vi "PicoScope2000ExampleBlockAdvancedTrigger.vi"() -> ()   [LabVIEW 2010]
uses:
  shared/PicoBuffers.ctl
  shared/Buffer and Transfer Settings.ctl
  shared/Acquisition Settings.ctl
  PicoScope2000Lib/PicoScope2000AnalogChannelSettings.ctl
panel:
  in  "Write to TDMS":bool
  in  "roundFaster":bool=TRUE
  in  "timeIntervalRequested":dbl min=0.0 format="%#6_6p"
  in  "Trigger Conditions":T1 {"PWQ" items=["Don't Care", "True", "False"]; "Ext" items=["Don't Care", "True", "False"]; "Channel D" items=["Don't Care", "True", "False"]; "Channel C" items=["Don't Care", "True", "False"]; "Channel B" items=["Don't Care", "True", "False"]; "Channel A" items=["Don't Care", "True", "False"]; "Condition Logic" items=["AND", "OR", "XOR"]}
  in  "Channel A Trigger Properties":T2={"thresholdUpper"=0, "thresholdHysteresis"=512, "thresholdLower"=0, "Threshold Mode"=0, "Direction"=2, "Available"=TRUE} {"Direction" items=["Above / Inside", "Below / Outside", "Rising / Enter", "Falling / Exit", "Rising or Falling / Enter or Exit", "Above Lower", "Below Lower", "Rising Lower", "Falling Lower", "Positive Runt", "Negative Runt"]; "Threshold Mode" items=["Level", "Window"]}
  in  "Pulse Width Qualifier Settings":T3={"Direction"=2, "Lower Limit"=0, "Upper Limit"=0, "Pulse Width Type"=0} {"Pulse Width Type" items=["None", "Less Than", "Greater Than", "In Range", "Out of Range"]; "Direction" items=["Rising"=2, "Falling"=3]}
  in  "Pulse Width Qualifier Conditions":T4 {"Condition Logic" items=["AND", "OR", "XOR"]}
  in  "Auto Trigger (ms)":i32=1000
  in  "Trigger Delay":u32
  in  "Channel B Settings":T5={"Enabled"=TRUE, "Coupling"=1, "Range"=6} {"Range" items=["20 mV"=1, "50 mV"=2, "100 mV"=3, "200 mV"=4, "500 mV"=5, "1 V"=6, "2 V"=7, "5 V"=8, "10 V"=9, "20 V"=10]; "Coupling" items=["AC", "DC"]}
  in  "Channel A Settings":T5={"Enabled"=TRUE, "Coupling"=1, "Range"=6} {"Range" items=["20 mV"=1, "50 mV"=2, "100 mV"=3, "200 mV"=4, "500 mV"=5, "1 V"=6, "2 V"=7, "5 V"=8, "10 V"=9, "20 V"=10]; "Coupling" items=["AC", "DC"]}
  out "Unit Info":T6
  out "overflow":i16 format="%010b"
  in  "Apply Settings":bool
  out "error out":errorcluster
  in  "Data file":path=path "PicoScope2000ExampleBlockAdvTrig Data"
  in  "Buffer and Transfer Settings":T7={"startIndex"=0, "Samples"=3968, "Down Sample Ratio"=1, "Down-Sample Mode"=0} {"Down-Sample Mode" items=["RAW none"=2147483648, "None"=0, "Aggregate"=1, "Decimate"=2, "Average"=4]; "Down Sample Ratio" step=1; "Samples" format="%_6p"}
  in  "Acquisition Settings":T8={"preTriggerSamples"=0, "postTriggerSamples"=3968, "timebase"=0} {"postTriggerSamples" format="%_6p"; "preTriggerSamples" format="%_6p"}
  out "Properties Panel":T9={"Sample Frequency"=3125000.0, "Sample Rate"=3.199999980552093e-07, "Max Samples Available"=3968, "Number of Samples"=3000, "Total Capture Time (sec) "=0.0009599999757483602, "Max Total Capture Time Available (sec)"=0.0012697599595412612} {"Max Total Capture Time Available (sec)" format="%.3p"; "Sample Frequency" format="%.6p"; "Sample Rate" format="%.3p"; "Max Samples Available" format="%_6p"; "Total Capture Time (sec)" format="%.3p"}
  in  "stop":bool
  out "Analog Channels":cluster{i32, dbl, "Data":dbl[]}[](graph)
  in  "error in (no error)":errorcluster
  # "For Condition Logic Suggested settings;\nFor AND, XOR logic-(parallel triggers)\nUse level-type triggers (Level or Inside/outside Window Triggers)\n\nFor OR logic- (single channel)\nUse edge types (e.g. rising, falling, entering window)"
  # "Bit 0 = ChA"
  # "Oversample control ->"
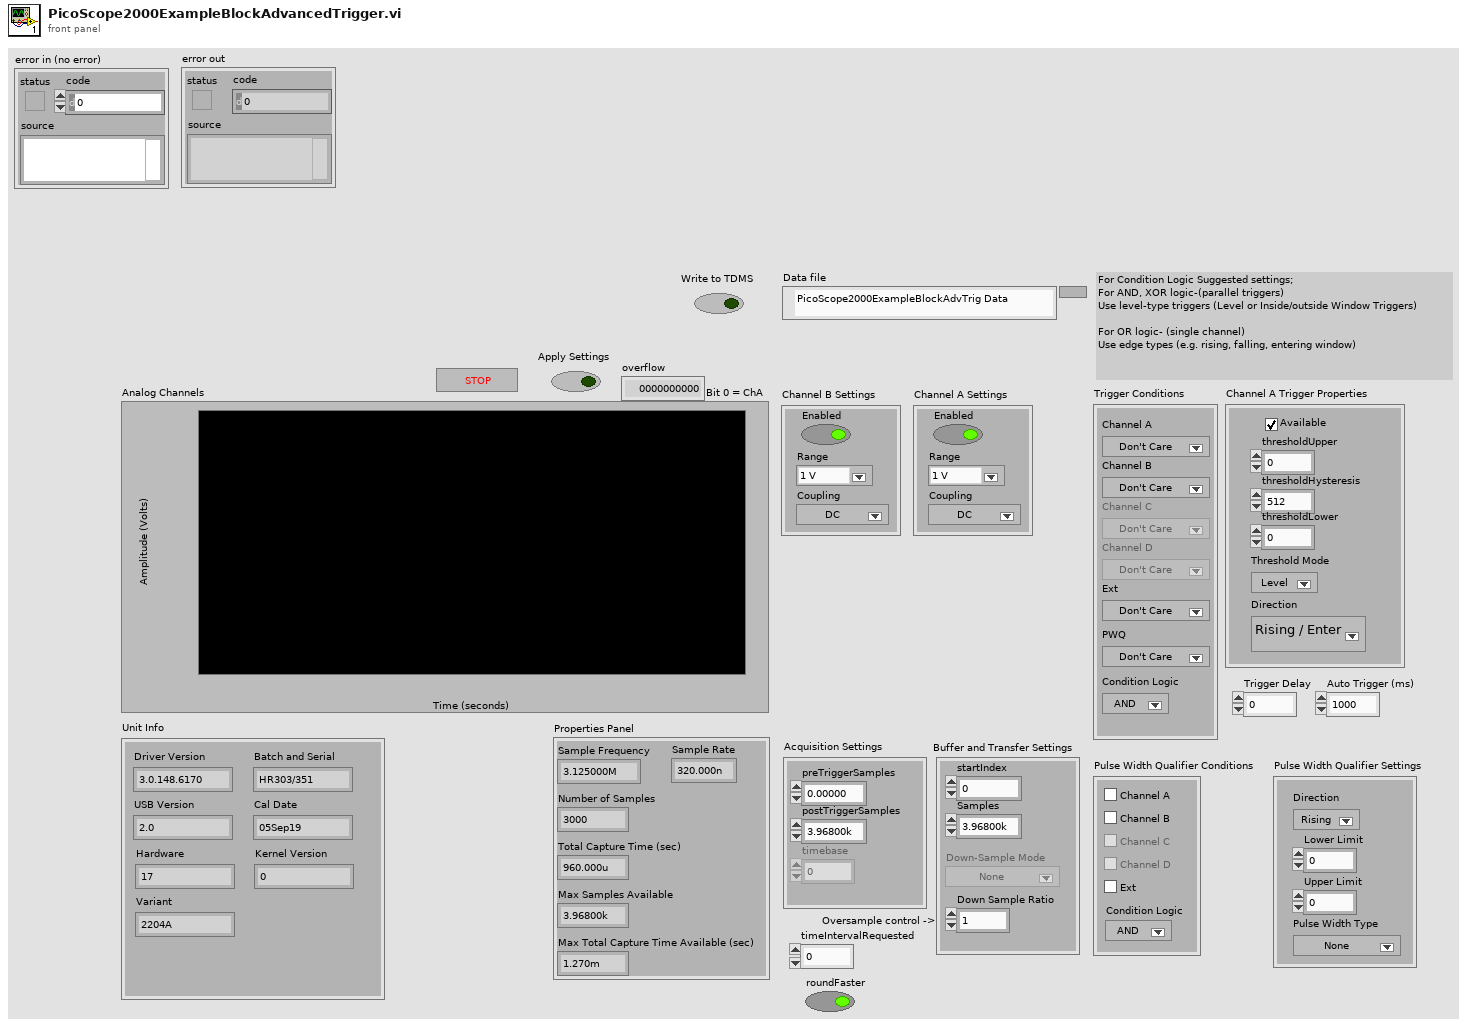
[diagram p1: front panel]
types:
  T1 = cluster{"Channel A":u16, "Channel B":u16, "Channel C":u16, "Channel D":u16, "Ext":u16, "PWQ":u16, "Condition Logic":u16}
  T2 = cluster{"thresholdUpper":i16, "thresholdHysteresis":u16, "thresholdLower":i16, "Threshold Mode":i32, "Direction":i32, "Available":bool}
  T3 = cluster{"Direction":u32, "Lower Limit":u32, "Upper Limit":u32, "Pulse Width Type":u32}
  T4 = cluster{"Channel A":bool, "Channel B":bool, "Channel C":bool, "Channel D":bool, "Condition Logic":u16, "Ext":bool}
  T5 = typedef "PicoScope2000AnalogChannelSettings.ctl" = cluster{"Enabled":bool, "Coupling":i16, "Range":u16}
  T6 = cluster{"Driver Version":string, "USB Version":string, "Hardware":string, "Variant":string, "Batch and Serial":string, "Cal Date":string, "Kernel Version":string}
  T7 = typedef "Buffer and Transfer Settings.ctl" = cluster{"startIndex":u64, "Samples":u64, "Down Sample Ratio":u64, "Down-Sample Mode":u32}
  T8 = typedef "Acquisition Settings.ctl" = cluster{"preTriggerSamples":u64, "postTriggerSamples":u64, "timebase":u32}
  T9 = cluster{"Sample Frequency":dbl, "Sample Rate":dbl, "Max Samples Available":u64, "Number of Samples":u64, "Total Capture Time (sec) ":dbl, "Max Total Capture Time Available (sec)":dbl}
  T10 = typedef "PicoBuffers.ctl" = cluster{"Max Buffer Pointers":u64[][][], "Min Buffer Pointers":u64[][][], "StreamingDataInfo":cluster{"Channel":u32, "Down-Sample Mode":u32, "PICO_DATA_TYPE":enum32{"PICO_INT8_T", "PICO_INT16_T", "PICO_INT32_T", "PICO_UINT32_T", "PICO_INT64_T", ""}, "Samples":i32, "bufferIndex":u64, "startIndex":i32, "overflow":i16}[][]}
  T11 = enum16{"open", "open or create", "create or replace", "create", "open (read-only)"}
  T12 = cluster{"Sample Frequency":sgl, "Sample Rate":sgl, "Max Samples Available":i32, "Number of Samples":u32, "Total Capture Time (sec) ":sgl, "Max Total Capture Time Available (sec)":sgl}
  T13 = cluster{"Channel A Buffer":i16[], "Channel B Buffer":i16[], "Channel C Buffer":i16[], "Channel D Buffer":i16[], "Channel E Buffer":i16[], "Channel F Buffer":i16[], "Channel G Buffer":i16[], "Channel H Buffer":i16[], "Port 0 Buffer":i16[], "Port 1 Buffer":i16[]}[]
  T14 = cluster{"Channel A Buffer":i16[], "Channel B Buffer":i16[], "Channel C Buffer":i16[], "Channel D Buffer":i16[], "Channel E Buffer":i16[], "Channel F Buffer":i16[], "Channel G Buffer":i16[], "Channel H Buffer":i16[], "Port 0 Buffer":i16[], "Port 1 Buffer":i16[]}
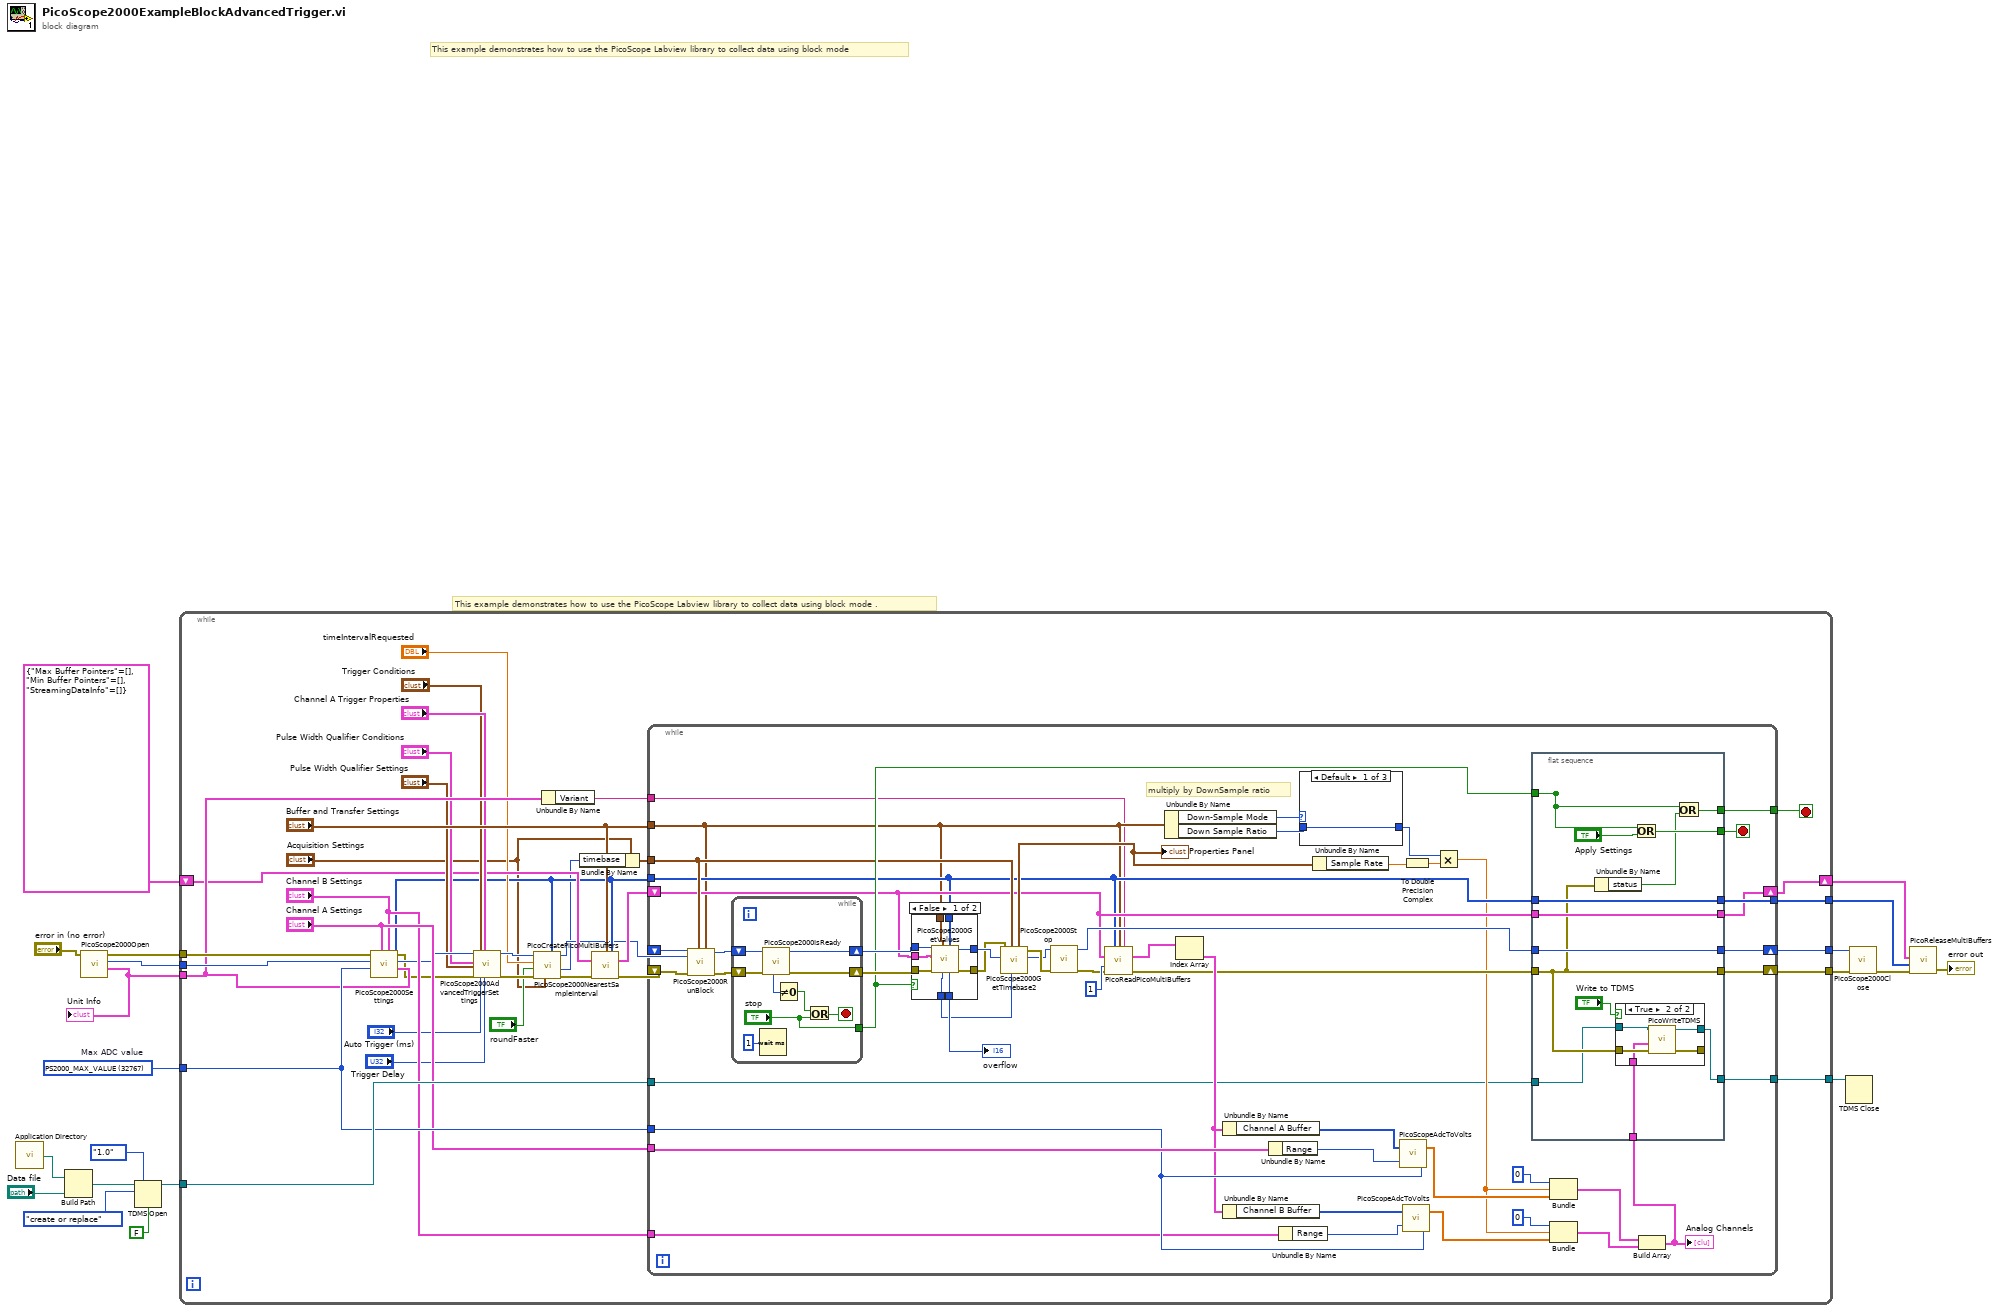
[diagram p0: block diagram]
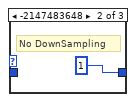
[diagram p4: hidden frame]
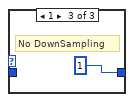
[diagram p5: hidden frame]
diagram:
  w3 = i16 32767 items=["PS2000_MAX_VALUE"=32767]  # Max ADC value
  # "This example demonstrates how to use the PicoScope Labview library to collect data using block mode ."
  # "This example demonstrates how to use the PicoScope Labview library to collect data using block mode"
  n1 = call <vilib>:"Application Directory.vi"() -> ("Application Directory"=w14:path)
  n2 = Build Path(base path=w14, name or relative path="Data file") -> (appended path=w15:path)
  n3 = call "PicoScope2000Open.vi"("error in (no error)"="error in (no error)") -> ("Unit Info"=w6:T6, "handle"=w7:i16, "error out"=w8:errorcluster)  [unwired: 6 in]
  "Unit Info" <- w6
  n4 = TDMS Open(6:FALSE ("disable buffering? (T)"), 7:enum16{"1.0", "2.0"}."1.0" ("file format version (2.0)"), 10:T11."create or replace" ("operation (0:open)"), 11:w15) -> (3:w12:refnum<k34>)  [unwired: 2 in, 1 out]
  n5 = while {
    tunnel: w7 -> [w54]
    tunnel: w3 -> [w48]
    tunnel: [w42] -> w20
    tunnel: [w51] -> w13
    tunnel: w12 -> [w55]
    tunnel: w6 -> [w47]
    tunnel: w8 -> [w53]
    tunnel: [w52] -> w4
    tunnel: [w49] -> w5
    shift-right: [w31] -> w1
    shift-left: T10 {"Max Buffer Pointers"=[], "Min Buffer Pointers"=[], "StreamingDataInfo"=[]} ("Data Pointers") -> [w32]
    stop <- w50 stop-if-true
    n6 = call "PicoScope2000Settings.vi"("Unit Info"=w47, "Channel B Settings"="Channel B Settings", "Channel A Settings"="Channel A Settings", "Max ADC value"=w48, "handle in"=w54, "error in"=w53) -> ("Enabled Array"=w26:i16[], "handle out"=w41:i16, "error out"=w40:errorcluster)  [unwired: 1 in]
    n7 = call "PicoScope2000AdvancedTriggerSettings.vi"("handle in"=w41, "Pulse Width Qualifier Conditions"="Pulse Width Qualifier Conditions", "Pulse Width Qualifier Settings"="Pulse Width Qualifier Settings", "error in"=w40, "Trigger Conditions"="Trigger Conditions", "Auto Trigger (ms)"="Auto Trigger (ms)", "Channel A Trigger Properties"="Channel A Trigger Properties", "Trigger Delay"="Trigger Delay") -> ("handle out"=w28:i16, "error out"=w30:errorcluster)  [unwired: 10 in]
    n8 = call "PicoScope2000NearestSampleInterval.vi"("Enabled Array"=w26, "Acquisition Settings"="Acquisition Settings", "error in (no error)"=w30, "roundFaster"="roundFaster", "timeIntervalRequested"="timeIntervalRequested", "handle in"=w28) -> ("error out"=w29:errorcluster, "timebase"=w21:i16, "handle out"=w24:i16)  [unwired: 2 in, 1 out]
    n9 = Unbundle By Name(w47) -> ("Variant"=w33:string)
    n10 = Bundle By Name(cluster="Acquisition Settings", "timebase"=w21) -> (w23:T8)
    n11 = call "PicoCreatePicoMultiBuffers.vi"("Buffer and Transfer Settings"="Buffer and Transfer Settings", "enabled array"=w26, "Data Pointers In"=w32, "error in (no error)"=w29) -> ("Data Pointers"=w56:T10, "error out"=w45:errorcluster)  [unwired: 10 in]
    n12 = while {
      tunnel: "Buffer and Transfer Settings" -> [w72]
      tunnel: w26 -> [w74]
      tunnel: "Channel A Settings" -> [w104]
      tunnel: w23 -> [w80]
      tunnel: w48 -> [w103]
      tunnel: [w89] -> w50
      shift-right: [w91] -> w52
      shift-left: w45 -> [w68]
      shift-right: [w87] -> w49
      shift-left: w24 -> [w67]
      tunnel: w55 -> [w59]
      tunnel: [w60] -> w51
      tunnel: "Channel B Settings" -> [w81]
      tunnel: [w75] -> w42
      tunnel: w33 -> [w71]
      shift-right: [w69] -> w31
      shift-left: w56 -> [w76]
      stop <- w88 stop-if-true
      # "multiply by DownSample ratio"
      n13 = call "PicoScope2000RunBlock.vi"("Buffer and Transfer Settings"=w72, "Acquisition Settings"=w80, "error in (no error)"=w68, "handle in"=w67) -> ("error out"=w106:errorcluster, "handle out"=w105:i16)  [unwired: 4 in, 2 out]
      n14 = while {
        shift-right: [w148] -> w85
        shift-left: w106 -> [w149]
        shift-right: [w147] -> w86
        shift-left: w105 -> [w146]
        tunnel: ["stop"] -> w84
        stop <- w143 stop-if-true
        n15 = Wait (ms)(milliseconds to wait=u32 1) -> ()  [unwired: 1 out]
        n16 = call "PicoScope2000IsReady.vi"("error in (no error)"=w149, "handle in"=w146) -> ("error out"=w148:errorcluster, "handle out"=w147:i16, "ready"=w145:i16)  [unwired: 7 in]
        n17 = Not Equal To 0?(x=w145) -> (x != 0?=w144:bool)
        n18 = Or(x=w144, y="stop") -> (x .or. y?=w143:bool)
      }
      n19 = case shown="False" w84 {
        tunnel: w85 -> [w118 w119]
        tunnel: w86 -> [w117 w120]
        tunnel: [w116 w120] -> w65
        tunnel: [w115 w119] -> w64
        tunnel: [w114 _] -> w83
        tunnel: [w113 _] -> w66
        tunnel: w74 -> [w112 _]
        tunnel: w76 -> [w111 _]
        tunnel: w72 -> [w110 _]
        frame False {
          n20 = call "PicoScope2000GetValues.vi"("enabled array"=w112, "Buffer and Transfer Settings"=w110, "error in (no error)"=w118, "Data Pointers In"=w111, "handle in"=w117) -> ("error out"=w115:errorcluster, "handle out"=w116:i16, "overflow"=w114:i16, "noOfSamples"=w113:u64)  [unwired: 3 in]
        }
        frame True {
        }
      }
      "overflow" <- w83
      n21 = call "PicoScope2000GetTimebase2.vi"("Memory Segment"=w66, "Acquisition Settings"=w80, "handle in"=w65, "error in (no error)"=w64) -> ("handle out"=w62:i16, "error out"=w63:errorcluster, "Properties Panel"=w79:T12)  [unwired: 5 in]
      "Properties Panel" <- w79
      n22 = call "PicoScope2000Stop.vi"("error in (no error)"=w63, "handle in"=w62) -> ("error out"=w78:errorcluster, "handle out"=w77:i16)  [unwired: 8 in]
      n23 = call "PicoReadPicoMultiBuffers.vi"("enabled array"=w74, "Buffer and Transfer Settings"=w72, "Variant"=w71, "Data Pointers"=w76, "No of Buffers"=1, "error in (no error)"=w78) -> ("MultiBuffers (Max or non-aggregated)"=w109:T13, "error out"=w90:errorcluster)  [unwired: 7 in, 1 out]
      n24 = Unbundle By Name(w72) -> ("Down-Sample Mode"=w107:u32, "Down Sample Ratio"=w108:u64)
      n25 = Index Array(array=w109) -> (element=w92:T14)  [unwired: 1 in]
      n26 = Unbundle By Name(w92) -> ("Channel A Buffer"=w93:i16[])
      n27 = Unbundle By Name(w92) -> ("Channel B Buffer"=w98:i16[])
      n28 = Unbundle By Name(w104) -> ("Range"=w100:u16)
      n29 = Unbundle By Name(w81) -> ("Range"=w82:u16)
      n30 = case shown="Default" w107 {
        tunnel: [w150 u64 1 ("Down Sample Ratio") u64 1 ("Down Sample Ratio")] -> w73
        tunnel: w108 -> [w150 _ _]
        frame Default {
        }
        frame -2147483648 {
          # "No DownSampling"
        }
        frame 1 {
          # "No DownSampling"
        }
      }
      n31 = Unbundle By Name(w79) -> ("Sample Rate"=w58:sgl)
      n32 = call "PicoScopeAdcToVolts.vi"("Max_adc"=w103, "Range Index"=w100, "Data"=w93) -> ("Data"=w94:dbl[])
      n33 = call "PicoScopeAdcToVolts.vi"("Max_adc"=w103, "Range Index"=w82, "Data"=w98) -> ("Data"=w97:dbl[])
      n34 = To Double Precision Complex(1:w58) -> (0:w57:cdb)
      n35 = Multiply(x=w73, y=w57) -> (x*y=w70:cdb)
      n36 = flat-sequence {
        tunnel: [w133] -> w88
        tunnel: [w128] -> _
        tunnel: [w130] -> w89
        tunnel: w77 -> [w129]
        tunnel: [w129] -> w87
        tunnel: w90 -> [w124]
        tunnel: [w124] -> w91
        tunnel: w84 -> [w128]
        tunnel: w76 -> [w127]
        tunnel: [w127] -> w69
        tunnel: [w126] -> w75
        tunnel: w74 -> [w126]
        tunnel: w61 -> [w123]
        tunnel: [w122] -> w60
        tunnel: w59 -> [w121]
        frame #0 {
          n37 = Unbundle By Name(w124) -> ("status"=w131:bool)
          n38 = case shown="True" "Write to TDMS" {
            tunnel: [w135 w140] -> w122
            tunnel: [w134 w139] -> _
            tunnel: w124 -> [w134 w138]
            tunnel: w123 -> [_ w137]
            tunnel: w121 -> [w135 w136]
            frame False {
            }
            frame True {
              n39 = call "PicoWriteTDMS.vi"("error in (no error)"=w138, "Analog Channels"=w137, "Refnum in"=w136) -> ("error out"=w139:errorcluster, "Refnum out"=w140:refnum<k34>)  [unwired: 7 in]
            }
          }
          n40 = Or(x=w128, y="Apply Settings") -> (x .or. y?=w133:bool)
          n41 = Or(x=w128, y=w131) -> (x .or. y?=w130:bool)
        }
      }
      n42 = Bundle(0, w70, "Data"=w94) -> (w96:cluster{i32, cdb, "Data":dbl[]})  [unwired: 1 in]
      n43 = Bundle(0, w70, "Data"=w97) -> (w95:cluster{i32, cdb, "Data":dbl[]})  [unwired: 1 in]
      n44 = Build Array(w96, w95) -> (w61:cluster{i32, cdb, "Data":dbl[]}[])
      "Analog Channels" <- w61
    }
  }
  n45 = TDMS Close(11:w13) -> ()  [unwired: 1 in, 2 out]
  n46 = call "PicoScope2000Close.vi"("error in"=w4, "handle"=w5) -> ("error out"=w9:errorcluster)  [unwired: 4 in, 1 out]
  n47 = call "PicoReleaseMultiBuffers.vi"("error in (no error)"=w9, "Enabled array"=w20, "Data Pointers"=w1) -> ("error out"=→"error out":errorcluster)  [unwired: 7 in, 1 out]
